vi "AlazarFFTSetup.vi"(0 "DSP Handle":u64, 1 "Input Channel Mask":u16(ring)=1 items=["CHANNEL_A"=1], 2 "Record Length (samples)":u32, 3 "FFT Length (samples)":u32, 4 "Output Format":u32(ring)=1 items=["U32_AMP2"=0, "U16_LOG"=1, "U16_AMP2"=257, "U8_LOG"=2, "U8_AMP2"=258, "REAL_S32"=3, "IMAG_S32"=4, "FLOAT_AMP2"=10, "FLOAT_LOG"=11, "RAW_PLUS_FFT"=4096], 5 "Footer":u32(ring) items=["FOOTER_NONE", "FOOTER_NPT"], 6 "Reserved":u32, 7 "error in (no error)":errorcluster) -> (20 "DSP Handle":u64, 21 "Bytes Per Output Record":u32, 26 "Return Code":u32, 27 "error out":errorcluster)   [LabVIEW 2018]
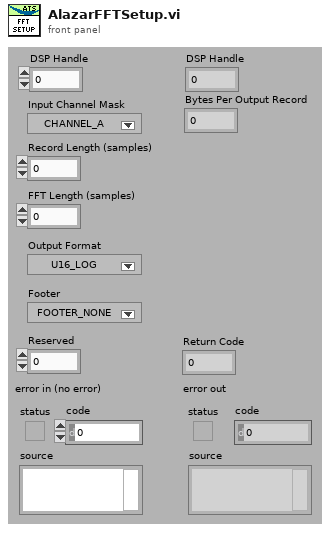
[diagram p1: front panel]
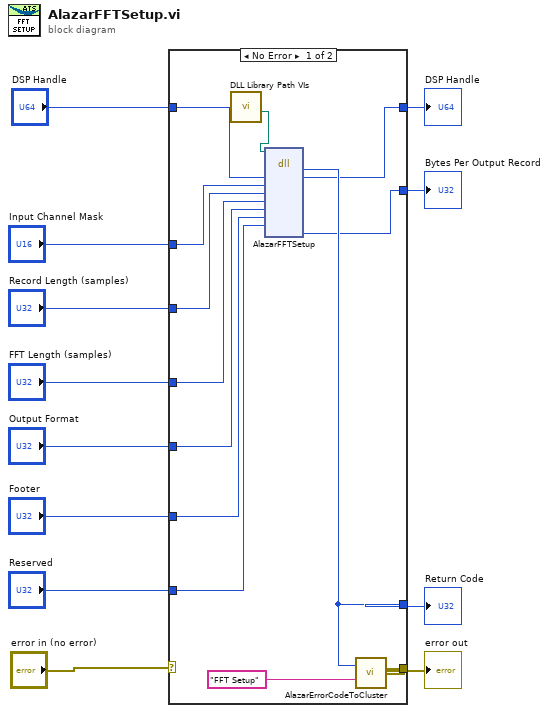
[diagram p0: block diagram]
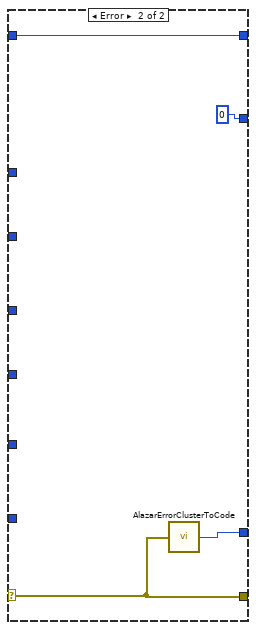
[diagram p2: hidden frame]
diagram:
  n1 = case shown="No Error" "error in (no error)" {
    selector: "error in (no error)" -> [_ w29]
    tunnel: [w22 w29] -> w11
    tunnel: [w24 w28] -> w10
    tunnel: "DSP Handle" -> [w25 w27]
    tunnel: [w21 w27] -> w8
    tunnel: "Input Channel Mask" -> [w20 _]
    tunnel: "Record Length (samples)" -> [w19 _]
    tunnel: "FFT Length (samples)" -> [w18 _]
    tunnel: "Output Format" -> [w17 _]
    tunnel: "Footer" -> [w16 _]
    tunnel: "Reserved" -> [w15 _]
    tunnel: [w14 0] -> w1
    frame No Error {
      n2 = call "DLL Library Path VIs.vi"() -> ("Alazar"=w13:path)  [unwired: 5 in, 6 out]
      n3 = dll-call lib="C:/Project/SerialSectOCT - FFT GPU/SerialSectOCT/Labview Software/DLL/ATSApi.dll" fn="AlazarFFTSetup"(path in=w13, "handle"=w25, "inputChannelMask"=w20, "recordLength_samples"=w19, "fftLength_samples"=w18, "outputFormat"=w17, "footer"=w16, "reserved"=w15) -> ("return type"=w24:u32, "handle"=w21:u64, "bytesPerOutputRecord"=w14:u32)  [unwired: 9 in, 2 out]
      n4 = call "AlazarErrorCodeToCluster.vi"("Message"="FFT Setup", "Error Code"=w24) -> ("error out"=w22:errorcluster)
    }
    frame Error {
      n5 = call "AlazarErrorClusterToCode.vi"("error in (no error)"=w29) -> ("Error Code"=w28:u32)
    }
  }
  "DSP Handle" <- w8
  "error out" <- w11
  "Return Code" <- w10
  "Bytes Per Output Record" <- w1
